vi "custom_1_stimulus_advanced.vi"(3 "Input Array":dbl[](array[numeric]), 4 "Input AFG Settings":dbl[][](array[numeric])=[[0.0, 100.0, 1.0]], 5 "Cluster":T1) -> (0 "x != y?":bool, 1 "Output Array":dbl[](array[numeric]), 2 "Output AFG Settings":dbl[][](array[numeric]))   [LabVIEW 2010]
panel:
  in  "Custom 1 stimulus duration (ms)":i32[][](array[numeric]) min=4 max=65535
  in  "Fraction of time between is active":dbl[][](array[numeric]) min=0.006818182300776243
  in  "stop":bool
  in  "OK Button":bool
  in  "Custom Stimulus Timing Array":dbl[](array[numeric])
  # "Duty Cycle"
  # "Switch time(ms)"
  # "Stimulus Timing Settings"
  # "Signal Duration Settings"
  # "Custom Stimulus Timing Array (ms)"
  # "Trigger signal duration (ms)"
  # "Switch time(ms)"
  # "AFG Settings"
  # "Amplitude(v)"
  # "Time (ms)"
  # "Frequency (Hz)"
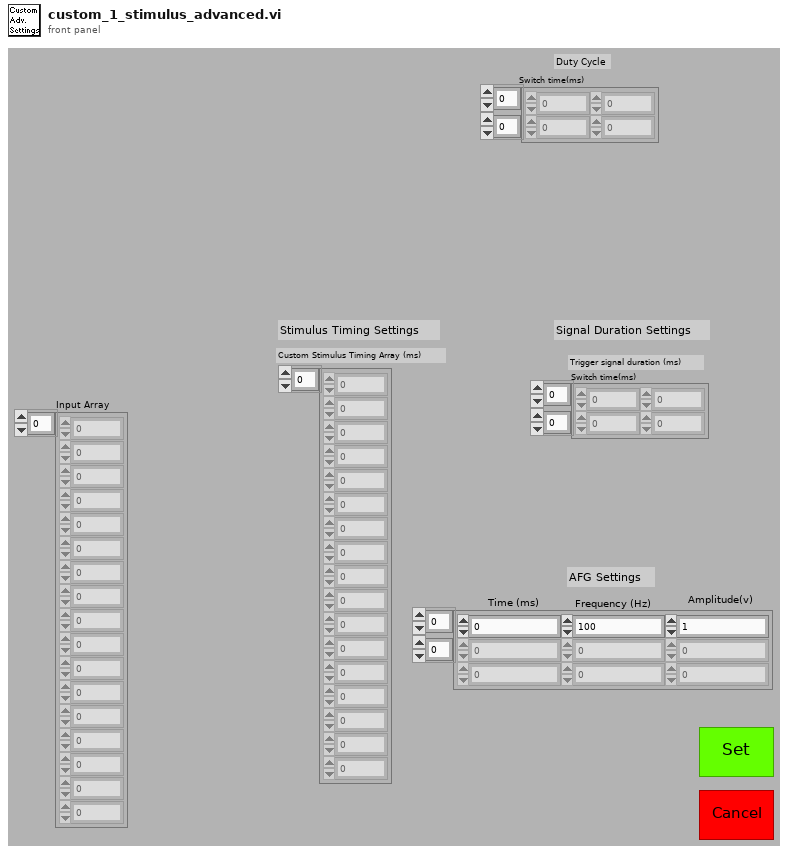
[diagram p1: front panel]
types:
  T1 = cluster{"custom 1 fraction of time between is active":refnum<vi>, "time between custom 1 onset":refnum<vi>}
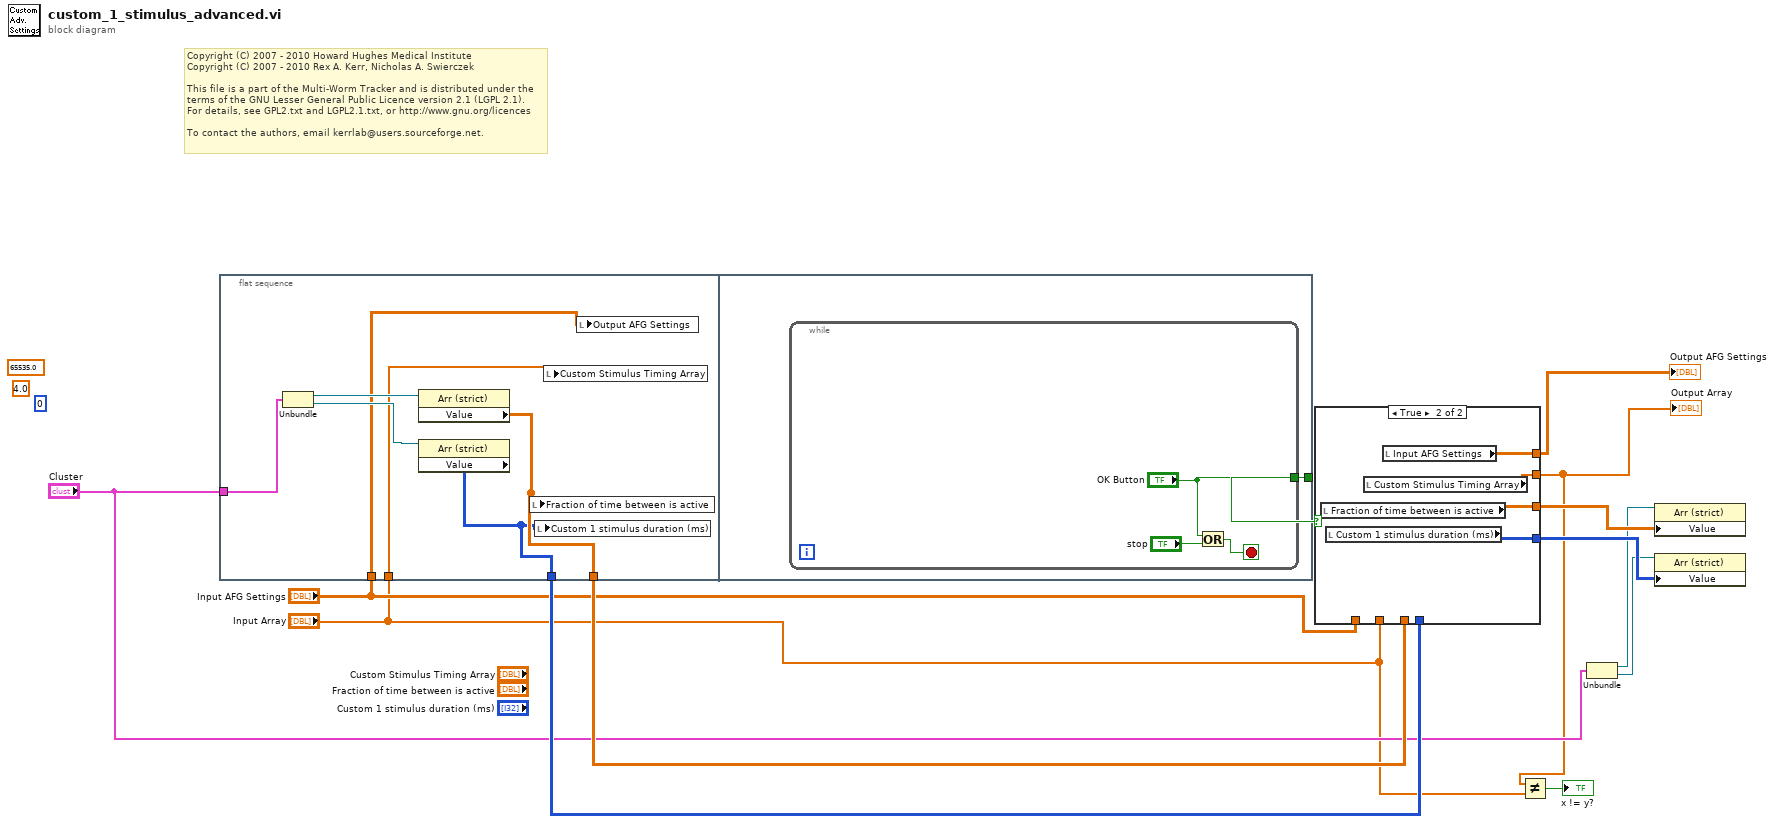
[diagram p0: block diagram]
diagram:
  (unwired) u8 0 ("Response to Value Outside Limits:Maximum")
  (unwired) 65535.0 ("x")
  (unwired) 4.0 ("Data Entry Limits:Minimum")
  # "Copyright (C) 2007 - 2010 Howard Hughes Medical Institute\nCopyright (C) 2007 - 2010 Rex A. Kerr, Nicholas A. Swierczek\n \nThis file is a part of the Multi-Worm Tracker and is distributed under the\nterms of the GNU Lesser General Public Licence version 2.1 (LGPL 2.1).\nFor details, see GPL2.txt and LGPL2.1.txt, or http://www.gnu.org/licences\n \nTo contact the authors, email kerrlab@users.sourceforge.net."
  n1 = flat-sequence {
    tunnel: "Cluster" -> [w19]
    tunnel: [w17] -> w7
    tunnel: [w16] -> w6
    tunnel: "Input AFG Settings" -> [w15]
    tunnel: "Input Array" -> [w14]
    tunnel: [w21] -> w13
    frame #0 {
      n2 = Unbundle(w19) -> ("custom 1 fraction of time between is active"=w18:refnum<vi>, "time between custom 1 onset"=w20:refnum<vi>)
      n3 = property class="Arr (strict)"(reference=w18) -> ("Value"=w17:sgl[][])  [unwired: 1 in, 2 out]
      n4 = property class="Arr (strict)"(reference=w20) -> ("Value"=w16:i32[][])  [unwired: 1 in, 2 out]
      n5 = local write "Fraction of time between is active"(w17) -> ()
      n6 = local write "Custom 1 stimulus duration (ms)"(w16) -> ()
      n7 = local write "Custom Stimulus Timing Array"(w14) -> ()
      n8 = local write "Output AFG Settings"(w15) -> ()
    }
    frame #1 {
      n9 = while {
        tunnel: ["OK Button"] -> w21
        stop <- w24 stop-if-true
        n10 = Or(x="OK Button", y="stop") -> (x .or. y?=w24:bool)
      }
    }
  }
  n11 = case shown="True" w13 {
    tunnel: "Input Array" -> [w28 _]
    tunnel: [w28 w32] -> w3
    tunnel: [w27 w31] -> w12
    tunnel: [w26 w30] -> w11
    tunnel: w7 -> [w27 _]
    tunnel: w6 -> [w26 _]
    tunnel: [w25 w29] -> w8
    tunnel: "Input AFG Settings" -> [w25 _]
    frame False {
    }
    frame True {
      n12 = local read "Fraction of time between is active"() -> (w31:dbl[][])
      n13 = local read "Custom 1 stimulus duration (ms)"() -> (w30:i32[][])
      n14 = local read "Custom Stimulus Timing Array"() -> (w32:dbl[])
      n15 = local read "Input AFG Settings"() -> (w29:dbl[][])
    }
  }
  "Output Array" <- w3
  "Output AFG Settings" <- w8
  n16 = Not Equal?(x=w3, y="Input Array") -> (x != y?=→"x != y?":bool)
  n17 = Unbundle("Cluster") -> ("custom 1 fraction of time between is active"=w10:refnum<vi>, "time between custom 1 onset"=w9:refnum<vi>)
  n18 = property class="Arr (strict)"(reference=w10, "Value"=w12) -> ()  [unwired: 1 in, 2 out]
  n19 = property class="Arr (strict)"(reference=w9, "Value"=w11) -> ()  [unwired: 1 in, 2 out]
